vi "FPGA_EventNodeTest.vi"() -> ()   [LabVIEW 2014]
uses:
  <vilib>/rvi/Emulation/niFpgaGetClockAttributes.vi
  <vilib>/rvi/Emulation/niFpgaSctlEmulationGetInTimedLoop.vi
  <vilib>/rvi/Emulation/niFpgaEmulationReportErrorSimple.vi
  <vilib>/rvi/occurrence/nirviWaitOnOccurrenceBase.vi
  <vilib>/rvi/Emulation/niFpgaCriticalErrorInLSC.vi
  <vilib>/rvi/Emulation/niFpgaProcessEmulError.vi
panel:
  in  "OK Button":bool
  out "Loop2":i16
  out "Loop1":i16
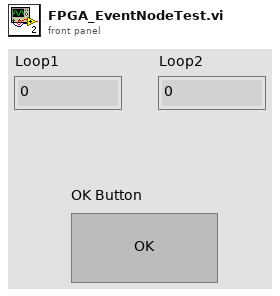
[diagram p1: front panel]
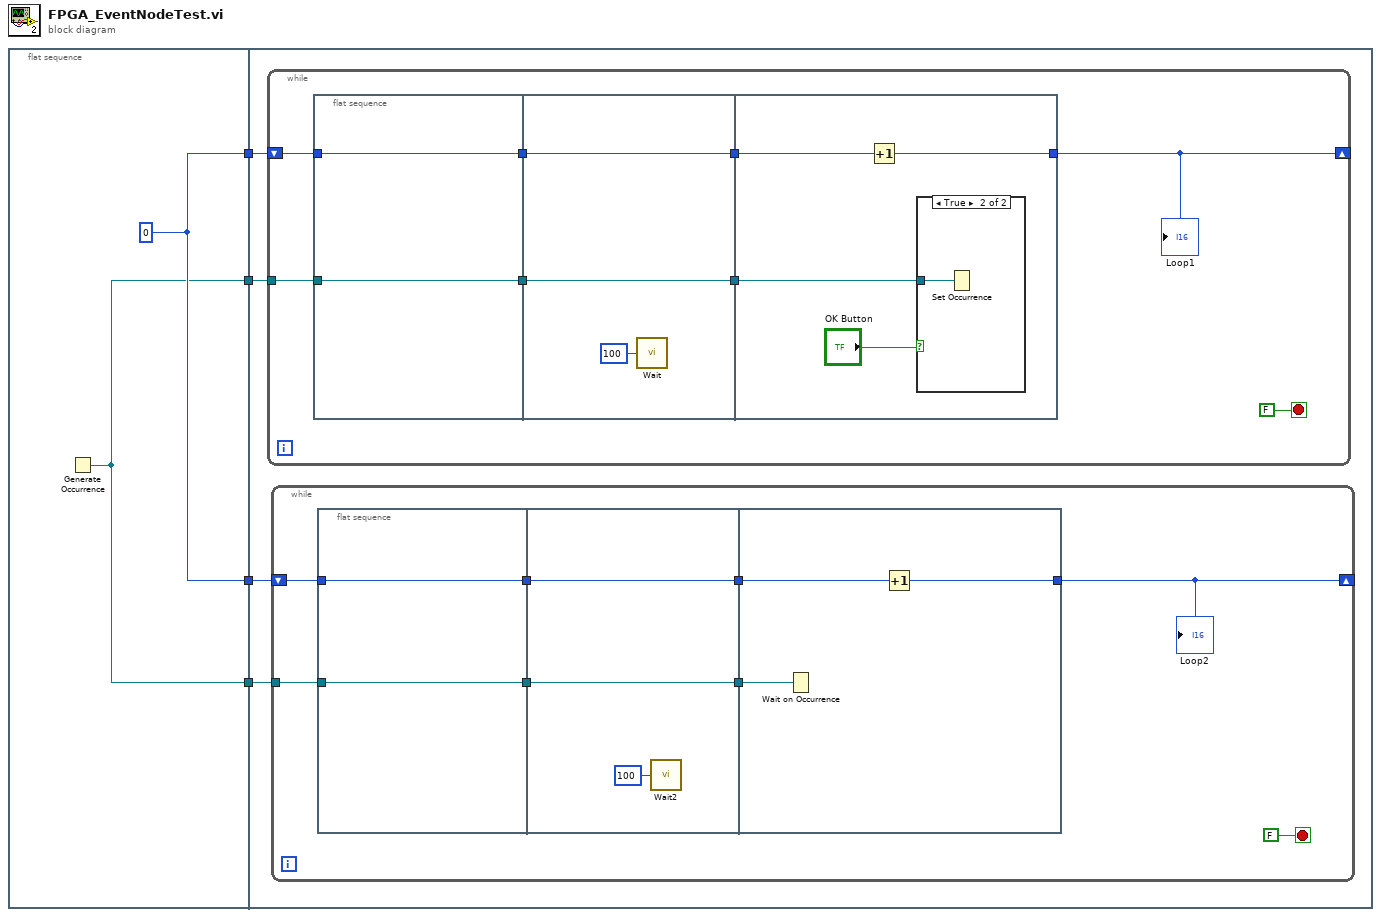
[diagram p0: block diagram]
diagram:
  n1 = flat-sequence {
    tunnel: [w6] -> w4
    tunnel: [w6] -> w3
    tunnel: [w5] -> w2
    tunnel: [w5] -> w1
    tunnel: w4 -> [w10]
    tunnel: w3 -> [w9]
    tunnel: w2 -> [w8]
    tunnel: w1 -> [w7]
    frame #0 {
      w6 = i16 0
      n2 = Generate Occurrence() -> (w5:refnum<k4>)
    }
    frame #1 {
      n3 = while {
        shift-right: [w31] -> _
        shift-left: w10 -> [w34]
        tunnel: w8 -> [w29]
        stop <- FALSE stop-if-true
        n4 = flat-sequence {
          tunnel: w34 -> [w36]
          tunnel: [w36] -> w32
          tunnel: w29 -> [w35]
          tunnel: [w35] -> w27
          tunnel: [w39] -> w33
          tunnel: w32 -> [w39]
          tunnel: [w37] -> w28
          tunnel: w27 -> [w37]
          tunnel: [w42] -> w31
          tunnel: w33 -> [w43]
          tunnel: w28 -> [w40]
          frame #0 {
          }
          frame #1 {
            n5 = call "Wait"("Count(mSec)"=u32 100) -> ()  [unwired: 1 out]
          }
          frame #2 {
            n6 = Increment(x=w43) -> (x+1=w42:i16)
            n7 = case shown="True" "OK Button" {
              tunnel: w40 -> [_ w44]
              frame False {
              }
              frame True {
                n8 = Set Occurrence(w44) -> ()
              }
            }
          }
        }
        "Loop1" <- w31
      }
      n9 = while {
        shift-right: [w15] -> _
        shift-left: w9 -> [w16]
        tunnel: w7 -> [w11]
        stop <- FALSE stop-if-true
        n10 = flat-sequence {
          tunnel: [w20] -> w17
          tunnel: w16 -> [w20]
          tunnel: [w19] -> w12
          tunnel: w11 -> [w19]
          tunnel: [w23] -> w18
          tunnel: w17 -> [w23]
          tunnel: [w21] -> w13
          tunnel: w12 -> [w21]
          tunnel: w18 -> [w26]
          tunnel: [w25] -> w15
          tunnel: w13 -> [w24]
          frame #0 {
          }
          frame #1 {
            n11 = call "Wait2"("Count(mSec)"=u32 100) -> ()  [unwired: 1 out]
          }
          frame #2 {
            n12 = Wait on Occurrence(2:w24) -> ()  [unwired: 2 in, 1 out]
            n13 = Increment(x=w26) -> (x+1=w25:i16)
          }
        }
        "Loop2" <- w15
      }
    }
  }
